vi "test random gaussian.vi"() -> ()   [LabVIEW 2021]
uses:
  <vilib>/Analysis/baseanly.llb/Mean (DBL).vi
  <vilib>/Analysis/NI_AALBase.lvlib
panel:
  out "Plot: circles":cluster{dbl[], dbl[]}(graph)
  in  "normalizatoon":dbl(slide)=4.0 scale=0.0..20.0
  in  "number of steps":i32(slide)=16 scale=0.0..1000.0
  in  "array lngth":i32=50
  out "variance":dbl format="%0.2f"
  out "standard deviation":dbl format="%0.2f"
  out "mean":dbl format="%0.2f"
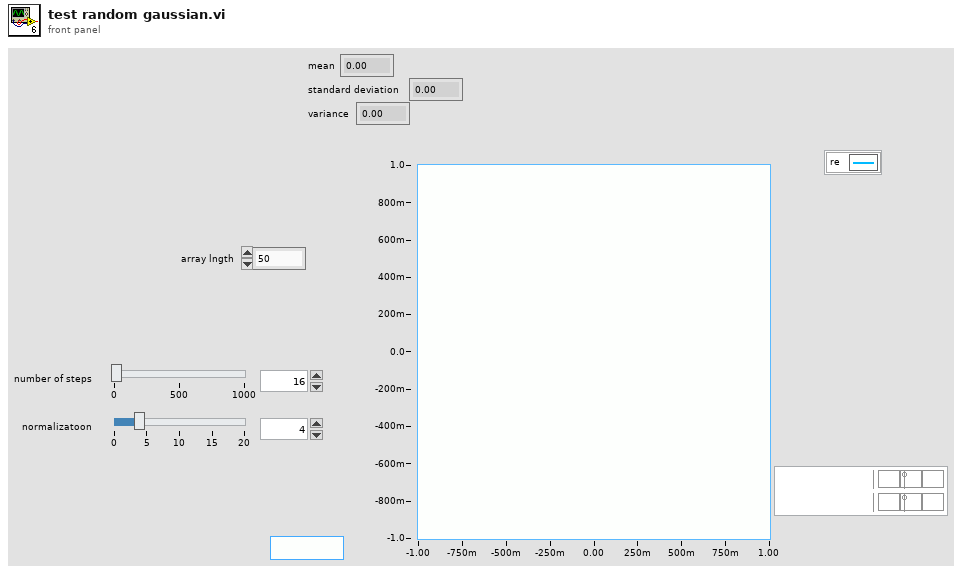
[diagram p1: front panel]
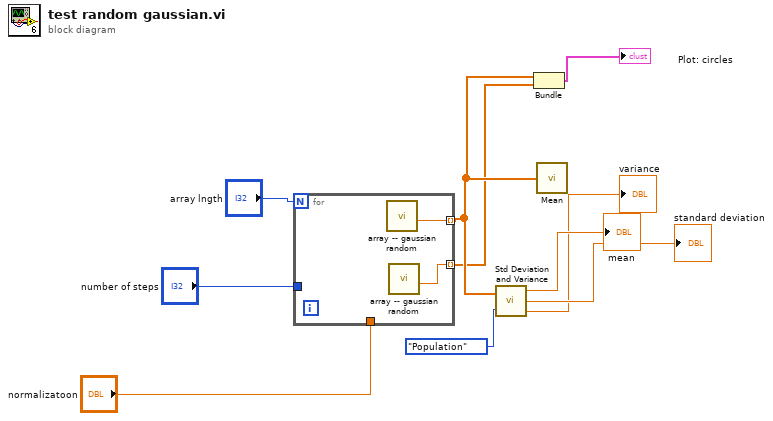
[diagram p0: block diagram]
diagram:
  n1 = for {
    N: "array lngth" -> [_]
    tunnel: [w12] -> w3 mode=indexing
    tunnel: "number of steps" -> [_]
    tunnel: "normalizatoon" -> [_]
    tunnel: [w11] -> w2 mode=indexing
    n2 = call "array -- gaussian random.vi"() -> ("number"=w12:dbl)  [unwired: 11 in]
    n3 = call "array -- gaussian random.vi"() -> ("number"=w11:dbl)  [unwired: 11 in]
  }
  n4 = call <vilib>:"Std Deviation and Variance.vi"("X"=w3, "Weighting (Sample)"=enum16{"Sample", "Population"}."Population") -> ("mean"=→"mean":dbl, "standard deviation"=→"standard deviation":dbl, "variance"=→"variance":dbl)
  n5 = Bundle(w3, w2) -> (→"Plot: circles":cluster{dbl[], dbl[]})  [unwired: 1 in]
  n6 = call-poly <vilib>:"Mean.vi"("X"=w3) -> ()  [unwired: 2 out]
